vi "OE2012&OE2022_Configure Auto Range.vi"(7 "OE2012&OE2022_\nAuto Range":T1={"Auto Gain"=FALSE, "Signal In Channel"=1} {"Signal In Channel" items=["Signal In 1"=1, "Signal In 2"=2]}, 8 "Error in (no error)":errorcluster caption="error out（no error）", 9 "Remote Mode":u16(ring) items=["USB", "RS232", "GPIB", "Ethernet"], 10 "Connection ID in":refnum<k5>, 11 "VISA resource name":refnum<visa-resource-name>) -> (0 "Error out":errorcluster caption="error out", 1 "Output String":string, 2 "Connection ID out":refnum<k5>, 3 "VISA resource  out":refnum<visa-resource-name>)   [LabVIEW 2011]
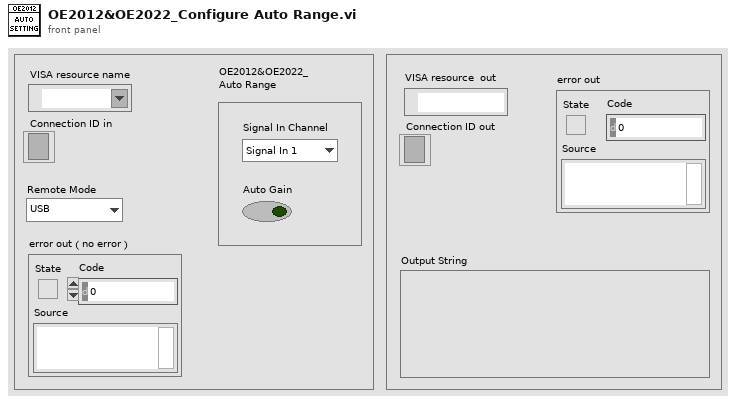
[diagram p1: front panel]
types:
  T1 = cluster{"Auto Gain":bool, "Signal In Channel":u16}
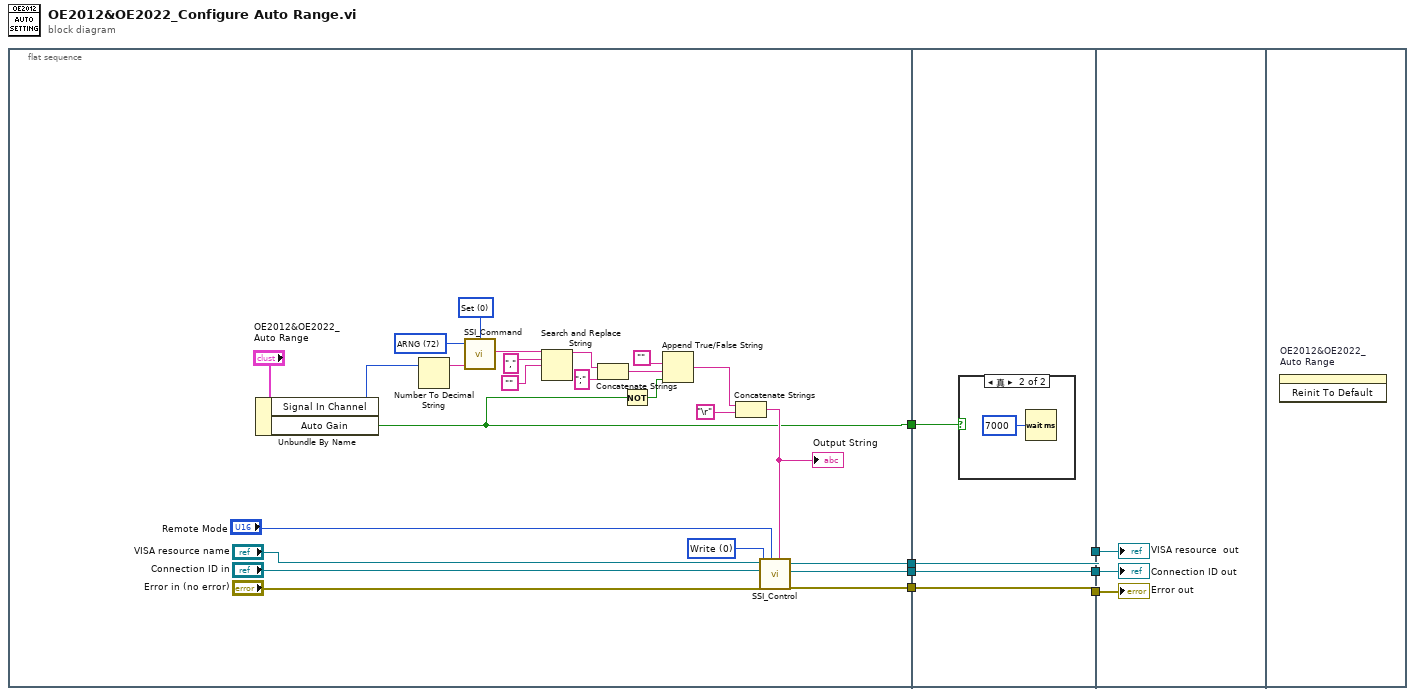
[diagram p0: block diagram]
diagram:
  n1 = flat-sequence {
    tunnel: [w28] -> w7
    tunnel: [w27] -> w6
    tunnel: [w26] -> w5
    tunnel: [w10] -> w1
    tunnel: w7 -> [w36]
    tunnel: w6 -> [w35]
    tunnel: w5 -> [w34]
    tunnel: [w36] -> w4
    tunnel: [w35] -> w3
    tunnel: [w34] -> w2
    tunnel: w1 -> [w33]
    tunnel: w4 -> [w39]
    tunnel: w3 -> [w40]
    tunnel: w2 -> [w38]
    frame #0 {
      w15 = u16 72 items=["ISRC", "IGND", "ICPL", "ILIN", "PHAS", "FMOD", "RSLP", "FREQ", "SWPT", "SLLM", "SULM", "SSLL", "SSLG", "STLM", "SWRM", "IRNG", "SENS", "RMOD", "OFLT", "OFSL", "SYNC", "DMOD", "HARM", "DARB", "SWVT", "SLVL", "SVLL", "SVUL", "SVSL", "SVSG", "SVTM", "SVRM", "RALL", "SNAP", "OUTP", "OAUX", "COUT", "CAUX", "COFP", "CEXP", "FPOP", "OEXP", "*IDN", "*RST", "OVLD", "INOV", "GNOV", "*PLL", "SSET", "RSET", "AGAN", "APHS", "ARSV", "ASCL", "EQCD", "EQCS", "SPED", "SRAT", "SLEN", "SSLE", "STRG", "SPRM", "STRD", "PAUS", "REST", "SPTS", "TRCA", "TEMP", "RSTU", "INHZ", "DEQU", "SADD", "ARNG", "CSPE", "ISRCD", "IGNDD", "ICPLD", "ILIND", "PHASD", "FMODD", "RSLPD", "FREQD", "SWPTD", "SLLMD", "SULMD", "SSLLD", "SSLGD", "STLMD", "SWRMD", "SENSD", "RMODD", "OFLTD", "OFSLD", "SYNCD", "HARMD", "EQCDD", "EQCSD", "SNAPD", "OUTPD", "SWVTD", "SLVLD", "SVLLD", "SVULD", "SVSLD", "SVSGD", "SVTMD", "SVRMD", "SVDCD", "ARSVD", "AGAND", "APHSD", "ASCLD", "FPOPD", "CAUXD", "OEXPD", "SPEDD", "SRATD", "SLEND", "SSLED", "STRGD", "SPRMD", "STRDD", "PAUSD", "RESTD", "SPTSD", "TRCAD", "*IDND", "*RSTD", "INOVD", "GNOVD", "*PLLD", "SSETD", "RSETD", "RALLD", "NIPA", "NSMA", "NGWA", "NMAC", "NMOD", "TRIG", "TRCB", "INHZD", "ISAMD", "IRAGD", "RRAGD", "SOFFD", "DMODD", "COUTD", "COFPD", "CEXPD", "ARNGD", "OAUXD", "TRIM", "SUITD", "SNHZD", "AOFSD", "RSRC", "FEXT", "FINT", "DSRC", "DARF", "DEAF", "DREF", "SSRC", "STTL", "SIGO", "SLVL", "SOFF", "SPHS", "TPHS", "SMOD", "MARF", "AMSR", "AMDP", "FMSR", "FMDV", "PMSR", "PMDV", "CHDC", "AUXV", "AFLT", "AOFP"] ("Command Type")
      w16 = u16 0 items=["Set", "Query"] ("Opera")
      w29 = u16 0 items=["Write", "Read"] ("Control")
      n2 = Unbundle By Name("OE2012&OE2022_\nAuto Range") -> ("Signal In Channel"=w9:u16, "Auto Gain"=w10:bool)
      n3 = Number To Decimal String(number=w9) -> (decimal integer string=w8:string)  [unwired: 1 in]
      n4 = call "SSI_Command.vi"("Opera"=w16, "Paramter"=w8, "Command Type"=w15) -> ("Output string"=w19:string)  [unwired: 1 in]
      n5 = Search and Replace String(input string=w19, search string="," ("搜索字符串"), replace string="") -> (result string=w21:string)  [unwired: 5 in, 3 out]
      n6 = Concatenate Strings(w21, ";") -> (w20:string)
      n7 = Not(x=w10) -> (.not. x?=w11:bool)
      n8 = Append True/False String(1:w11, 2:w20, 3:"") -> (0:w17:string)  [unwired: 1 in]
      n9 = Concatenate Strings(w17, "\r") -> (w12:string)
      "Output String" <- w12
      n10 = call "SSI_Control.vi"("Write Buffer"=w12, "Remote Mode"="Remote Mode", "Error in (no error)"="Error in (no error)", "Control"=w29, "Connection ID in"="Connection ID in", "VISA resource name"="VISA resource name") -> ("Error out"=w26:errorcluster, "Connection ID out"=w28:refnum<k5>, "VISA resource  out"=w27:refnum<visa-resource-name>)  [unwired: 2 in, 1 out]
    }
    frame #1 {
      n11 = case shown="真" w33 {
        frame False {
        }
        frame True {
          n12 = Wait (ms)(milliseconds to wait=u32 7000 ("等待时间（毫秒）")) -> ()  [unwired: 1 out]
        }
      }
    }
    frame #2 {
      "Error out" <- w38
      "Connection ID out" <- w39
      "VISA resource  out" <- w40
    }
    frame #3 {
      n13 = invoke on="OE2012&OE2022_\nAuto Range" class="Clust (严格)" method="Reinit To Default"() -> ()  [unwired: 3 in, 3 out]
    }
  }
